vi "LVObject to JSON.vi"(5 "enable LabVIEW extensions? (T)":bool=TRUE, 6 "Pretty Print?":bool, 7 "BlueJSONtext LVClass Serializer in":refnum<class "BlueJSONtext LVClass Serializer.lvclass">, 8 "error in (no error)":errorcluster, 10 "Object":refnum<class>) -> (0 "error out":errorcluster, 2 "<JSON>Object":string)   [LabVIEW 2019, in "BlueJSONTextSerializer.lvlib" / "BlueJSONtext LVClass Serializer.lvclass"]
uses:
  BlueJSONtext LVClass Serializer.lvclass
  <vilib>/JDP Science/JSONtext/LVClass Serializer/JSONtext LVClass Serializer.lvclass
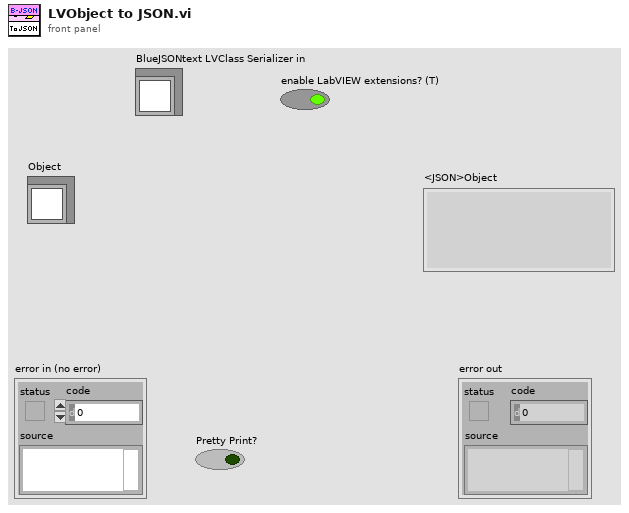
[diagram p1: front panel]
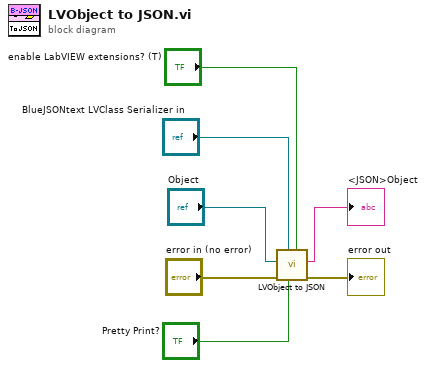
[diagram p0: block diagram]
diagram:
  n1 = call-parent "LVObject to JSON.vi"("enable LabVIEW extensions? (T)"="enable LabVIEW extensions? (T)", "Pretty Print?"="Pretty Print?", "JSONtext LVClass Serializer in"="BlueJSONtext LVClass Serializer in", "error in (no error)"="error in (no error)", "Object"="Object") -> ("error out"=→"error out":errorcluster, "<JSON>Object"=→"<JSON>Object":string)  [unwired: 5 in]
